vi "Str2DBL.vi"(5 "Error Locator":string, 6 "error in (no error)":errorcluster, 8 "Current Variable settings":T1[](array[typedef]), 9 "formula":string) -> (0 "error out":errorcluster, 3 "y value":dbl format="%#_15g")   [LabVIEW 2013]
doc: "Convert string to DBL. First try parsing with LuaVIEW \"Evaluate f(x)\", then scan for \"SI\" notation (e.g. 10u = 10e-5). Only white-space remainders allowed after the scan, otherwise an error is thrown. Output can be converted to boolean with \"!=0?\" comparison."
uses:
  TypeDefs/Active procedure variables.ctl
  <vilib>/Utility/error.llb/DialogType.ctl
panel:
  out "(Remainder String)":string
  out "(error lua)":errorcluster
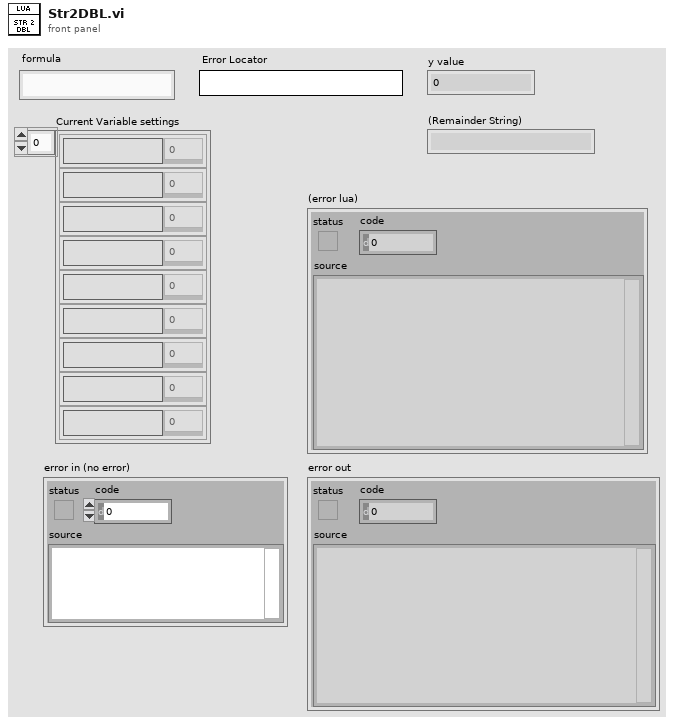
[diagram p1: front panel]
types:
  T1 = typedef "Active procedure variables.ctl" = cluster{"Procedure variable":string, "Value":dbl}
  T2 = typedef "DialogType.ctl" = u16
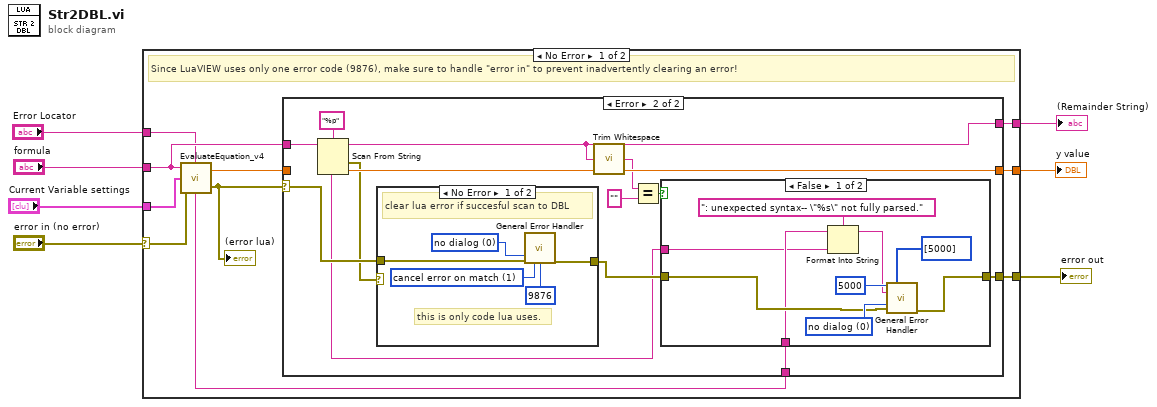
[diagram p0: block diagram]
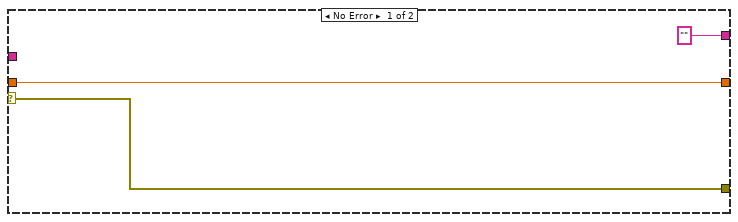
[diagram p2: hidden frame]
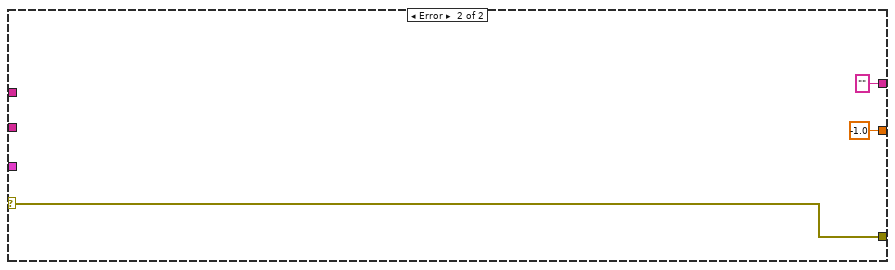
[diagram p5: hidden frame]
diagram:
  n1 = case shown="No Error" "error in (no error)" {
    selector: "error in (no error)" -> [w8 w50]
    tunnel: "Current Variable settings" -> [w16 _]
    tunnel: [w14 -1.0 ("y value")] -> w6
    tunnel: "formula" -> [w12 _]
    tunnel: [w11 w50] -> w4
    tunnel: "Error Locator" -> [w10 _]
    tunnel: [w9 ""] -> w2
    frame No Error {
      # "Since LuaVIEW uses only one error code (9876), make sure to handle \"error in\" to prevent inadvertently clearing an error!"
      n2 = call "EvaluateEquation_v4.vi"("Error Locator"=w10, "error in (no error)"=w8, "Current Variable settings"=w16, "formula"=w12) -> ("error out"=w15:errorcluster, "y value"=w13:dbl)
      "(error lua)" <- w15
      n3 = case shown="Error" w15 {
        selector: w15 -> [w18 w29]
        tunnel: [w19 w30] -> w14
        tunnel: w13 -> [w19 _]
        tunnel: w12 -> [_ w22]
        tunnel: [w18 w24] -> w11
        tunnel: w10 -> [_ w23]
        tunnel: ["" w20] -> w9
        frame No Error {
        }
        frame Error {
          n4 = Scan From String(format string="%p", input string=w22) -> (remaining string=w20:string, error out=w28:errorcluster, output 1=w30:dbl)  [unwired: 3 in, 1 out]
          n5 = case shown="No Error" w28 {
            tunnel: w29 -> [w46 w47]
            tunnel: [w45 w47] -> w25
            frame No Error {
              w42 = T2 0 items=["no dialog", "OK message", "continue or stop message", "OK message + warnings", "continue/stop + warnings"] ("type of dialog (OK msg:1)")
              w43 = 1 items=["no exception", "cancel error on match", "set error on match"] ("[exception action] (none:0)")
              # "this is only code lua uses."
              # "clear lua error if succesful scan to DBL"
              n6 = call <vilib>:"General Error Handler.vi"("type of dialog (OK msg:1)"=w42, "error in (no error)"=w46, "[exception action] (none:0)"=w43, "[exception code]"=9876) -> ("error out"=w45:errorcluster)  [unwired: 7 in, 4 out]
            }
            frame Error {
            }
          }
          n7 = call <vilib>:"Trim Whitespace.vi"("string"=w20) -> ("trimmed string"=w21:string)  [unwired: 1 in]
          n8 = Equal?(x=w21, y="") -> (x = y?=w26:bool)
          n9 = case shown="False" w26 {
            tunnel: w25 -> [w37 w41]
            tunnel: [w40 w41] -> w24
            tunnel: w23 -> [w35 _]
            tunnel: w22 -> [w32 _]
            frame False {
              w39 = T2 0 items=["no dialog", "OK message", "continue or stop message", "OK message + warnings", "continue/stop + warnings"] ("type of dialog (OK msg:1)")
              n10 = Format Into String(format string=": unexpected syntax-- \"%s\" not fully parsed.", initial string=w35, w32) -> (resulting string=w34:string)  [unwired: 1 in, 1 out]
              n11 = call <vilib>:"General Error Handler.vi"("[error code] (0)"=5000, "[user-defined codes]"=i32[] [5000], "[error source] (\" \")"=w34, "type of dialog (OK msg:1)"=w39, "error in (no error)"=w37) -> ("error out"=w40:errorcluster)  [unwired: 6 in, 4 out]
            }
            frame True {
            }
          }
        }
      }
    }
    frame Error {
    }
  }
  "y value" <- w6
  "error out" <- w4
  "(Remainder String)" <- w2
